vi "Write Set Load Control Msg.vi"(10 "Set Load Control Msg":refnum<class "Set Load Control Msg.lvclass">, 11 "SCADA Sub Abstract in":refnum<class "Device Communication and Control Abstract.lvclass">) -> (3 "SCADA Sub Abstract out":refnum<class "Device Communication and Control Abstract.lvclass">)   [LabVIEW 2018, in "Device Communication and Control Abstract Actor.lvlib" / "Device Communication and Control Abstract.lvclass"]
uses:
  Device Communication and Control Abstract.lvclass
  Device Communication and Control Abstract Messages/Set Load Control Msg/Set Load Control Msg.lvclass
  Device Communication and Control Abstract.lvclass/Device Communication and Control Abstract.ctl
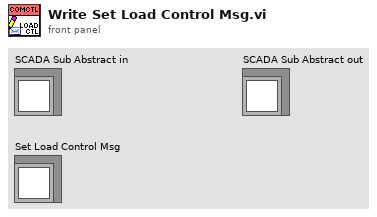
[diagram p1: front panel]
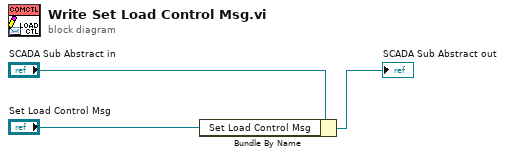
[diagram p0: block diagram]
diagram:
  n1 = Bundle By Name(cluster="SCADA Sub Abstract in", "Set Load Control Msg"="Set Load Control Msg") -> (→"SCADA Sub Abstract out":refnum<class "Device Communication and Control Abstract.lvclass">)
